vi "ConfigureSyringe.vi"(0 "object in":refnum<class "CetoniPump.lvclass">, 1 "index":i32, 2 "SyringeSettings":T1={"Maximum Piston Stroke (mm)"=100.0, "Inner Diameter (mm)"=12.0}, 5 "error in (no error)":errorcluster) -> (14 "object out":refnum<class "CetoniPump.lvclass">, 19 "error out":errorcluster)   [LabVIEW 2021, in "CetoniPump.lvclass"]
uses:
  CetoniPump.lvclass
  CetoniPump.lvclass/CetoniPump.ctl
  Users/olaja/AppData/Local/CETONI_SDK/lib/labview/labbCAN_Pump_API/labbCAN_Pump_API.lvlib
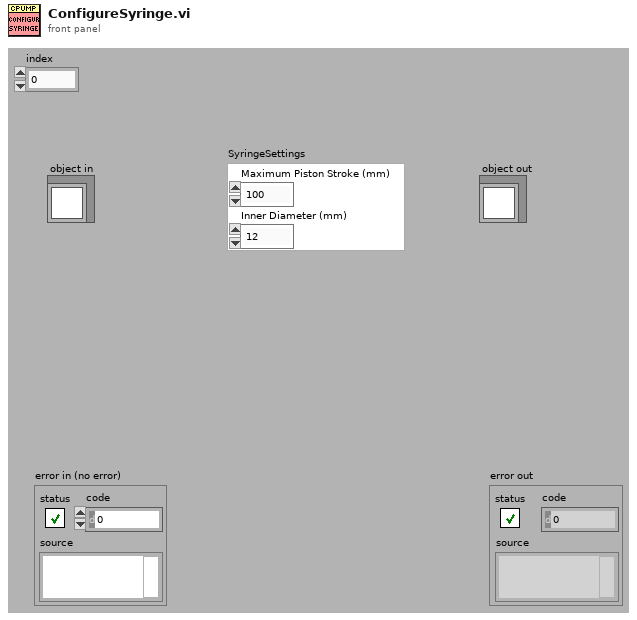
[diagram p1: front panel]
types:
  T1 = cluster{"Maximum Piston Stroke (mm)":dbl, "Inner Diameter (mm)":dbl}
  T2 = cluster{"Pump Handle":i64, "Pump Name":string, "Maximum Volume":dbl, "Maximum Flow Rate":dbl, "Flow Rate":dbl, "Target Level":dbl}[]
  T3 = cluster{"Pump Handle":i64, "Pump Name":string, "Maximum Volume":dbl, "Maximum Flow Rate":dbl, "Flow Rate":dbl, "Target Level":dbl}
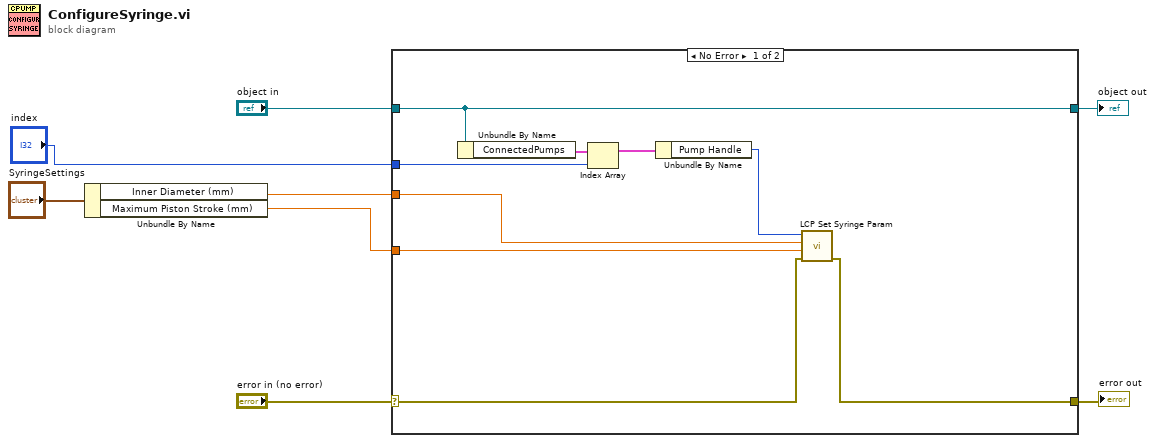
[diagram p0: block diagram]
diagram:
  n1 = Unbundle By Name("SyringeSettings") -> ("Inner Diameter (mm)"=w3:dbl, "Maximum Piston Stroke (mm)"=w2:dbl)
  n2 = case shown="No Error" "error in (no error)" {
    selector: "error in (no error)" -> [w14 w19]
    tunnel: [w15 w19] -> w7
    tunnel: [w17 w18] -> w5
    tunnel: "object in" -> [w17 w18]
    tunnel: w3 -> [w13 _]
    tunnel: w2 -> [w12 _]
    tunnel: "index" -> [w10 _]
    frame No Error {
      n3 = Unbundle By Name(w17) -> ("ConnectedPumps"=w16:T2)
      n4 = Index Array(array=w16, index=w10) -> (element=w11:T3)
      n5 = Unbundle By Name(w11) -> ("Pump Handle"=w9:i64)
      n6 = call "LCP Set Syringe Param.vi"("error in (no error)"=w14, "Maximum Piston Stroke (mm)"=w12, "Inner Diameter (mm)"=w13, "Pump Handle"=w9) -> ("error out"=w15:errorcluster)  [unwired: 7 in]
    }
    frame Error {
    }
  }
  "error out" <- w7
  "object out" <- w5
